vi "Add Files.vi"(8 "error in (no error)":errorcluster, 10 "Files":set{path}(c389), 11 "File Tree In":refnum<class "File Tree.lvclass">) -> (0 "error out":errorcluster, 3 "File Tree Out":refnum<class "File Tree.lvclass">)   [LabVIEW 2020, in "File Tree.lvclass"]
uses:
  File Tree.lvclass
  File Tree.lvclass/File Tree.ctl
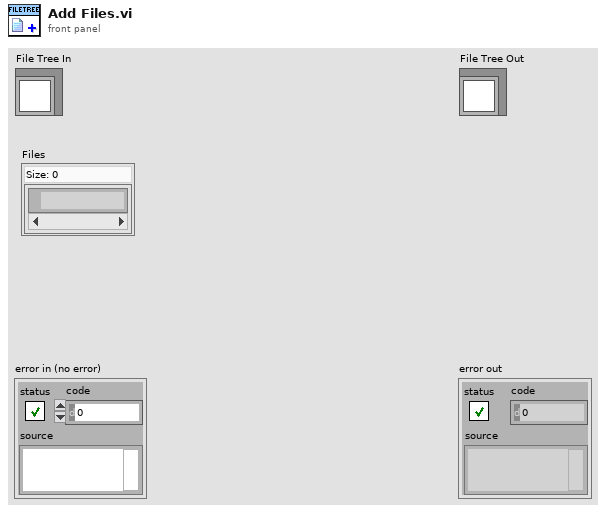
[diagram p1: front panel]
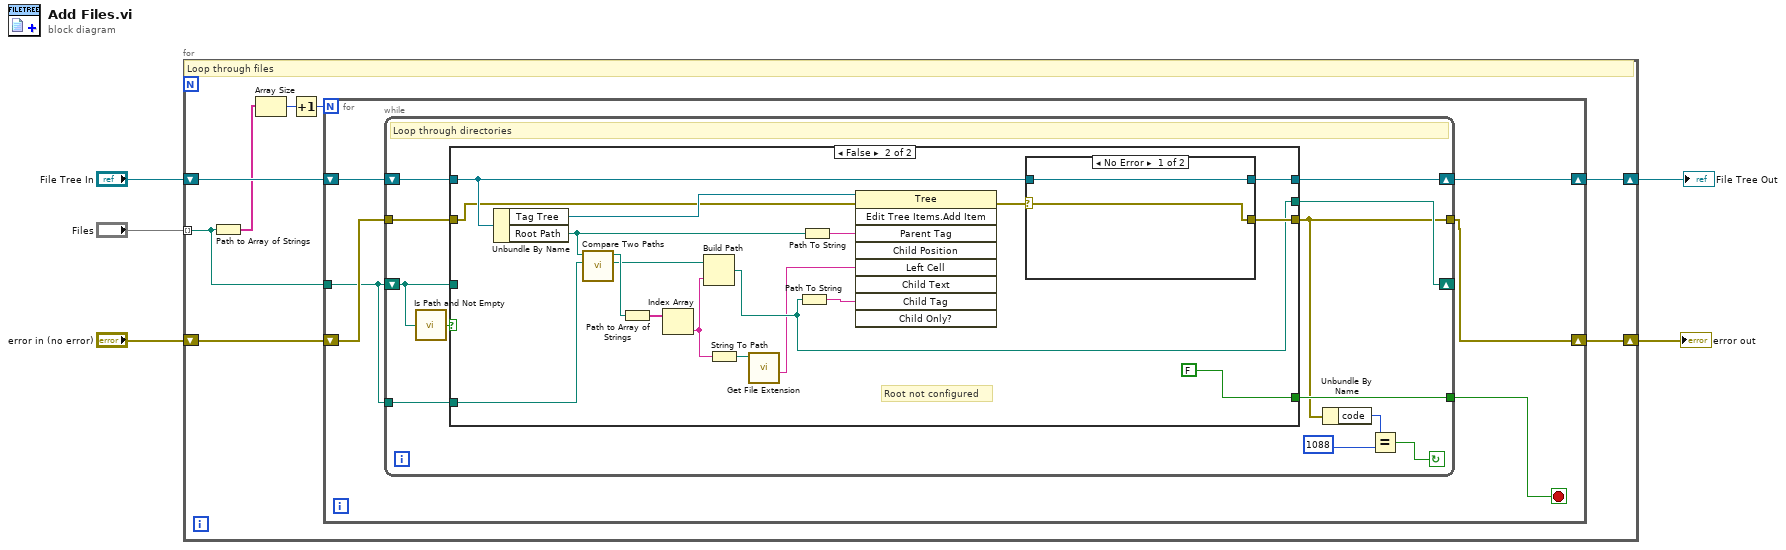
[diagram p0: block diagram]
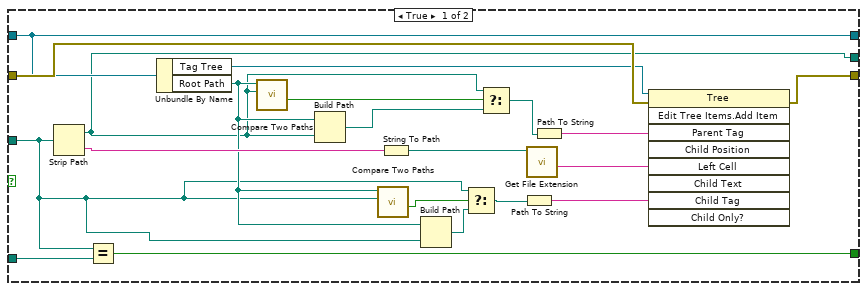
[diagram p2: hidden frame]
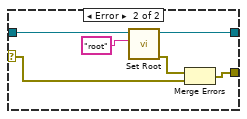
[diagram p3: hidden frame]
diagram:
  n1 = for {
    shift-right: [w13] -> w4
    shift-left: "File Tree In" -> [w12]
    shift-right: [w9] -> w5
    shift-left: "error in (no error)" -> [w10]
    tunnel: "Files" -> [w11] mode=indexing
    # "Loop through files"
    n2 = Path to Array of Strings(0:w11) -> (2:w8:string[])  [unwired: 1 out]
    n3 = Array Size(array=w8) -> (size(s)=w7:i32)
    n4 = Increment(x=w7) -> (x+1=w6:i32)
    n5 = for {
      N: w6 -> [_]
      tunnel: w11 -> [w16]
      shift-right: [w19] -> w13
      shift-left: w12 -> [w18]
      shift-right: [w14] -> w9
      shift-left: w10 -> [w17]
      stop <- w15 stop-if-true
      n6 = while {
        shift-right: [w26] -> w19
        shift-left: w18 -> [w31]
        shift-right: [w29] -> _
        shift-left: w16 -> [w28]
        tunnel: w17 -> [w30]
        tunnel: w16 -> [w25]
        tunnel: [w24] -> w15
        tunnel: [w20] -> w14
        stop <- w21 continue-if-true
        # "Loop through directories"
        n7 = call <vilib>:"Is Path and Not Empty.vi"("path"=w28) -> ("Is Path and Not Empty?"=w27:bool)  [unwired: 4 in]
        n8 = case shown="False" w27 {
          tunnel: w31 -> [w46 w66]
          tunnel: w30 -> [w48 w63]
          tunnel: [w47 w67] -> w20
          tunnel: [w35 w55] -> w29
          tunnel: w28 -> [w34 _]
          tunnel: [w46 w68] -> w26
          tunnel: w25 -> [w45 w59]
          tunnel: [w44 FALSE] -> w24
          frame True {
            n9 = Strip Path(path=w34) -> (stripped path=w35:path, name=w50:string)
            n10 = Equal?(x=w34, y=w45) -> (x = y?=w44:bool)
            n11 = Unbundle By Name(w46) -> ("Tag Tree"=w36:refnum<vi>, "Root Path"=w38:path)
            n12 = call <vilib>:"Compare Two Paths.vi"("Path 2"=w35, "Path 1"=w38) -> ("Path 2 Relative to Path 1?"=w43:bool)  [unwired: 6 in, 3 out]
            n13 = Build Path(base path=w38, name or relative path=w35) -> (appended path=w39:path)
            n14 = call <vilib>:"Compare Two Paths.vi"("Path 2"=w34, "Path 1"=w38) -> ("Path 2 Relative to Path 1?"=w42:bool)  [unwired: 6 in, 3 out]
            n15 = String To Path(string=w50) -> (path=w32:path)
            n16 = Build Path(base path=w38, name or relative path=w34) -> (appended path=w37:path)
            n17 = Select(t=w34, s=w42, f=w37) -> (s? t:f=w41:path)
            n18 = Select(t=w35, s=w43, f=w39) -> (s? t:f=w40:path)
            n19 = Path To String(path=w41) -> (string=w49:string)
            n20 = call <vilib>:"Get File Extension.vi"("file"=w32) -> ("filename without extension"=w33:string)  [unwired: 6 in, 4 out]
            n21 = Path To String(path=w40) -> (string=w51:string)
            n22 = invoke on="Invoke Node" class="Tree" method="Edit Tree Items.Add Item"(reference=w36, error in=w48, "Parent Tag"=w51, "Left Cell"=w33, "Child Tag"=w49) -> (error out=w47:errorcluster)  [unwired: 4 in, 8 out]
          }
          frame False {
            # "Root not configured"
            n23 = Unbundle By Name(w66) -> ("Tag Tree"=w65:refnum<vi>, "Root Path"=w60:path)
            n24 = call <vilib>:"Compare Two Paths.vi"("Path 2"=w59, "Path 1"=w60) -> ("Common Path"=w57:path, "Relative Path from 1 to 2"=w58:path)  [unwired: 6 in, 2 out]
            n25 = Path to Array of Strings(0:w58) -> (2:w56:string[])  [unwired: 1 out]
            n26 = Index Array(array=w56) -> (element=w53:string)  [unwired: 1 in]
            n27 = Build Path(base path=w57, name or relative path=w53) -> (appended path=w55:path)
            n28 = String To Path(string=w53) -> (path=w54:path)
            n29 = call <vilib>:"Get File Extension.vi"("file"=w54) -> ("filename without extension"=w52:string)  [unwired: 6 in, 4 out]
            n30 = Path To String(path=w55) -> (string=w61:string)
            n31 = Path To String(path=w60) -> (string=w62:string)
            n32 = invoke on="Invoke Node" class="Tree" method="Edit Tree Items.Add Item"(reference=w65, error in=w63, "Parent Tag"=w62, "Left Cell"=w52, "Child Tag"=w61) -> (error out=w64:errorcluster)  [unwired: 4 in, 8 out]
            n33 = case shown="No Error" w64 {
              selector: w64 -> [w70 w72]
              tunnel: [w71 w77] -> w68
              tunnel: [w70 w73] -> w67
              tunnel: w66 -> [w71 w74]
              frame No Error {
              }
              frame Error {
                n34 = call "Set Root.vi"("Root Name"="root", "File Tree In"=w74) -> ("error out"=w76:errorcluster, "File Tree Out"=w77:refnum<class "File Tree.lvclass">)  [unwired: 8 in]
                n35 = Merge Errors(w76, w72) -> (w73:errorcluster)
              }
            }
          }
        }
        n36 = Unbundle By Name(w20) -> ("code"=w23:i32)
        n37 = Equal?(x=w23, y=1088) -> (x = y?=w21:bool)
      }
    }
  }
  "error out" <- w5
  "File Tree Out" <- w4
